vi "Calculate String Info.vi"(0 "Str in":string, 5 "Str idx in":i32, 9 "Blob size in":i16[](array[numeric]), 11 "Blob elem in":i16[](array[numeric]), 13 "Is scalar":bool) -> (4 "Str out":string, 6 "Str idx out":i32)   [LabVIEW 2010]
doc: "See block diagram for VI documentation."
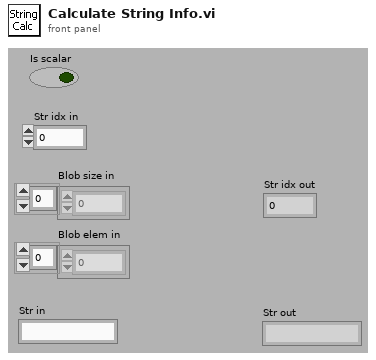
[diagram p1: front panel]
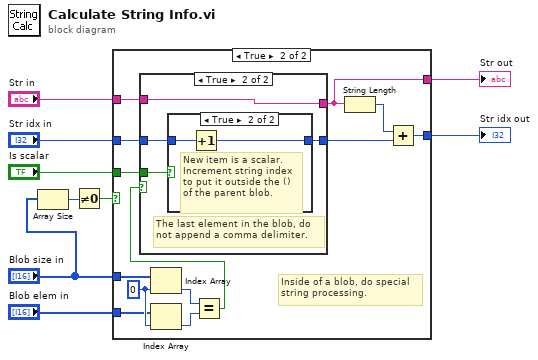
[diagram p0: block diagram]
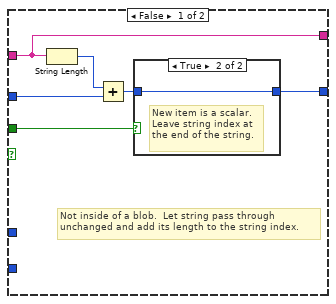
[diagram p2: hidden frame]
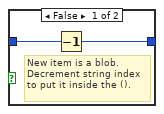
[diagram p3: hidden frame]
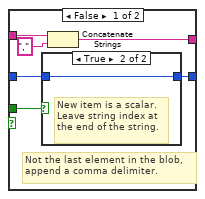
[diagram p4: hidden frame]
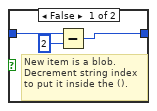
[diagram p5: hidden frame]
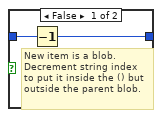
[diagram p6: hidden frame]
diagram:
  n1 = Array Size(array="Blob size in") -> (size(s)=w2:i32)
  n2 = Not Equal To 0?(x=w2) -> (x != 0?=w1:bool)
  n3 = case shown="True" w1 {
    tunnel: "Str in" -> [w13 w31]
    tunnel: "Str idx in" -> [w14 w28]
    tunnel: [w10 w29] -> w9
    tunnel: "Blob size in" -> [_ w24]
    tunnel: "Blob elem in" -> [_ w23]
    tunnel: "Is scalar" -> [w12 w20]
    tunnel: [w13 w19] -> w4
    frame False {
      (unwired) TRUE
      # "Not inside of a blob.  Let string pass through\nunchanged and add its length to the string index."
      n4 = String Length(string=w13) -> (length=w15:i32)
      n5 = Add(x=w15, y=w14) -> (x+y=w11:i32)
      n6 = case shown="True" w12 {
        tunnel: [w16 w18] -> w10
        tunnel: w11 -> [w17 w18]
        frame False {
          # "New item is a blob.\nDecrement string index\nto put it inside the ()."
          n7 = Decrement(x=w17) -> (x-1=w16:i32)
        }
        frame True {
          # "New item is a scalar.\nLeave string index at\nthe end of the string."
        }
      }
    }
    frame True {
      w26 = 0 ("index")
      # "Inside of a blob, do special\nstring processing."
      n8 = Index Array(array=w24, index=w26) -> (element=w21:i16)
      n9 = Index Array(array=w23, index=w26) -> (element=w22:i16)
      n10 = Equal?(x=w21, y=w22) -> (x = y?=w25:bool)
      n11 = case shown="True" w25 {
        tunnel: w31 -> [w37 w45]
        tunnel: [w35 w45] -> w19
        tunnel: w28 -> [w34 w44]
        tunnel: [w33 w43] -> w27
        tunnel: w20 -> [w32 w42]
        frame False {
          # "Not the last element in the blob,\nappend a comma delimiter."
          n12 = case shown="True" w32 {
            tunnel: [w38 w41] -> w33
            tunnel: w34 -> [w40 w41]
            frame False {
              # "New item is a blob.\nDecrement string index\nto put it inside the ()."
              n13 = Subtract(x=w40, y=2) -> (x-y=w38:i32)
            }
            frame True {
              # "New item is a scalar.\nLeave string index at\nthe end of the string."
            }
          }
          n14 = Concatenate Strings(w37, ",") -> (w35:string)
        }
        frame True {
          # "The last element in the blob, do\nnot append a comma delimiter."
          n15 = case shown="True" w42 {
            tunnel: w44 -> [w47 w49]
            tunnel: [w46 w48] -> w43
            frame False {
              # "New item is a blob.\nDecrement string index\nto put it inside the () but\noutside the parent blob."
              n16 = Decrement(x=w47) -> (x-1=w46:i32)
            }
            frame True {
              # "New item is a scalar.\nIncrement string index\nto put it outside the ()\nof the parent blob."
              n17 = Increment(x=w49) -> (x+1=w48:i32)
            }
          }
        }
      }
      n18 = String Length(string=w19) -> (length=w30:i32)
      n19 = Add(x=w30, y=w27) -> (x+y=w29:i32)
    }
  }
  "Str out" <- w4
  "Str idx out" <- w9
